vi "torque.vi"(5 "Optical":dbl, 6 "K":dbl=0.002, 7 "input_speed":dbl=905.26) -> (2 "Air gap distance":dbl, 3 "Torque":dbl format="%.5f")   [LabVIEW 2013]
panel:
  out "K 2":dbl
  in  "position":dbl[](array[numeric])=[0.006936158, 0.123434976, 0.06660524, 0.048499543, 0.042894394, 0.031233109, 0.017978293, -0.007572597, -0.007088973, -0.006314126, -0.013408862, -0.03698942, -0.059633605, -0.08709294, -0.061646755]
  in  "B":dbl[](array[numeric])=[361.6867357, 317.053774, 288.0813352, 251.2092617, 221.9672065, 202.0744938, 176.0201196, 159.6505095, 142.1246739, 127.4713834, 116.9721146, 102.8538267, 95.72786959, 84.33107726, 77.75646615]
  in  "Speed":dbl[](array[numeric])=[538.7343852, 571.7146956, 597.4120356, 616.9463637, 631.0607955, 641.0634852, 647.8692546, 652.8443821, 656.0759672, 658.4944862, 660.535588, 662.0915248, 663.3550631, 663.800211, 664.7743073]
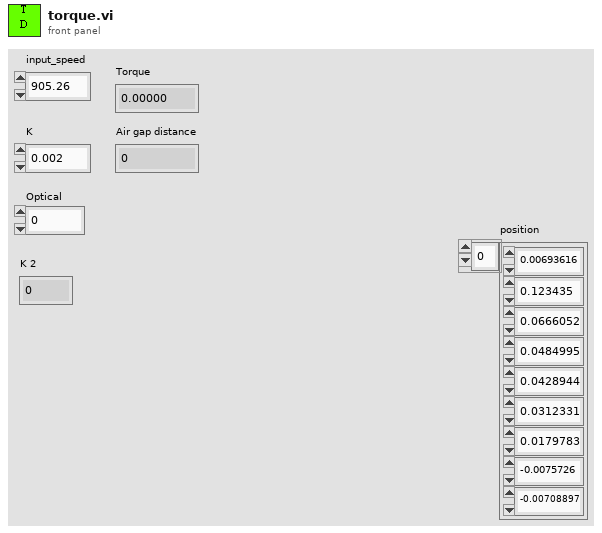
[diagram p1: front panel]
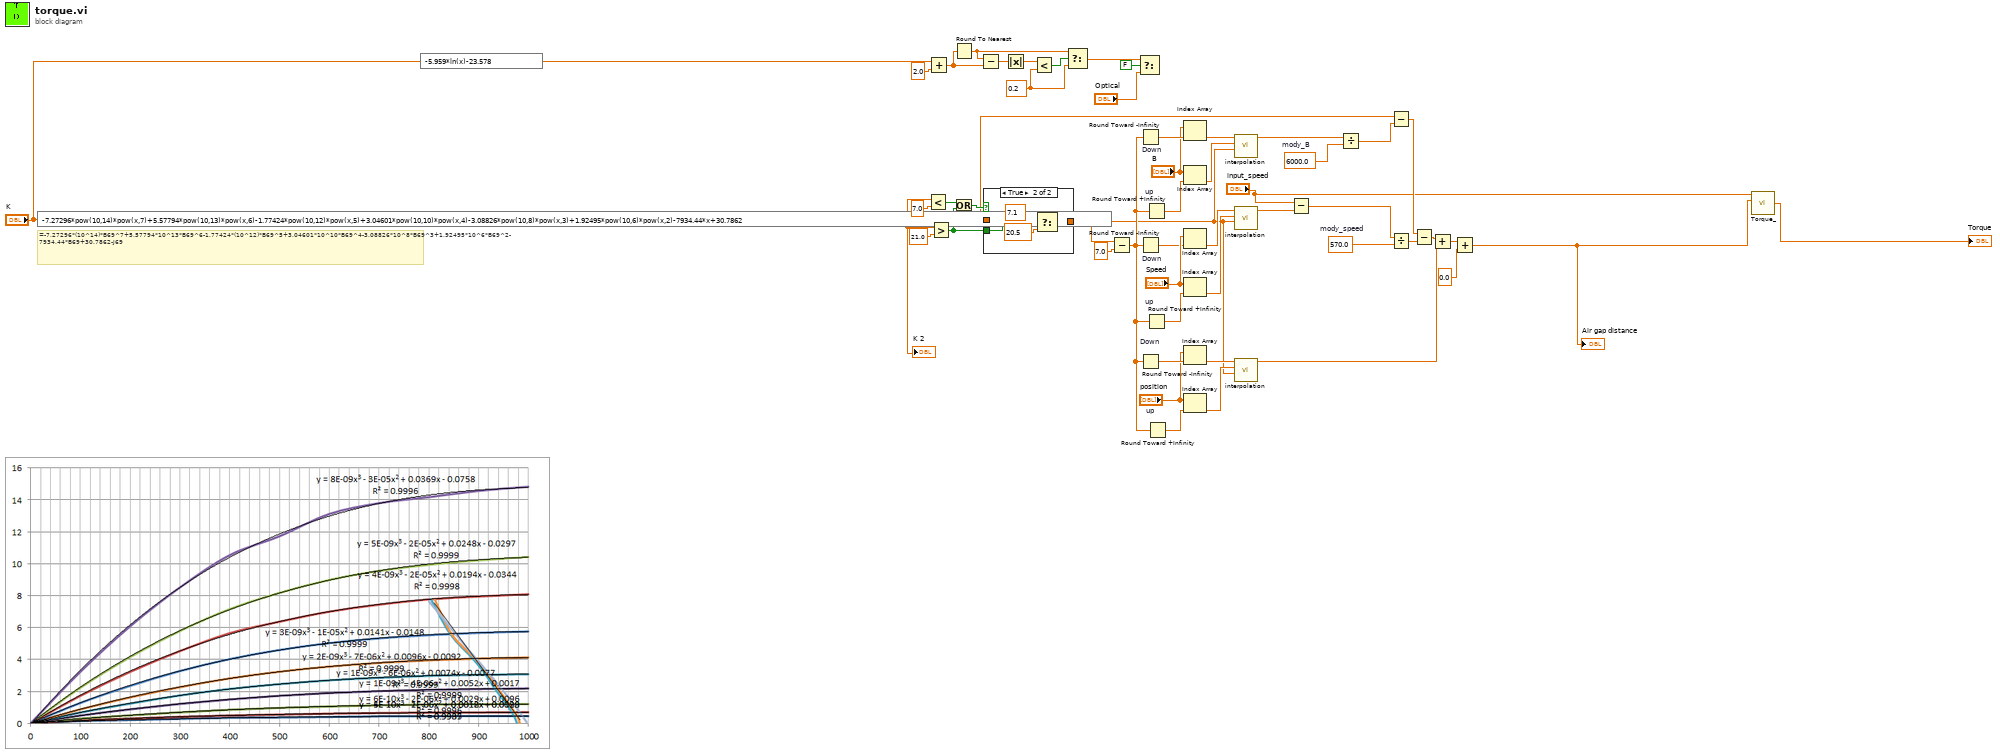
[diagram p0: block diagram]
diagram:
  w19 = 6000.0  # mody_B
  w26 = 570.0  # mody_speed
  w48 = 0.2 ("y")
  # "=-7.27296*(10^14)*B69^7+5.57794*10^13*B69^6-1.77424*(10^12)*B69^5+3.04601*10^10*B69^4-3.08826*10^8*B69^3+1.92495*10^6*B69^2-7934.44*B69+30.7862-J69"
  n1 = expression code="-7.27296*pow(10,14)*pow(x,7)+5.57794*pow(10,13)*pow(x,6)-1.77424*pow(10,12)*pow(x,5)+3.04601*pow(10,10)*pow(x,4)-3.08826*pow(10,8)*pow(x,3)+1.92495*pow(10,6)*pow(x,2)-7934.44*x+30.7862"("K") -> (w18:dbl)
  "K 2" <- w18
  n2 = expression code="-5.959*ln(x)-23.578"("K") -> (w47:dbl)
  n3 = Less?(x=w18, y=7.0) -> (x < y?=w35:bool)
  n4 = Add(x=w47, y=2.0) -> (x+y=w44:dbl)
  n5 = Greater?(x=w18, y=21.0) -> (0:w33:bool)
  n6 = Round To Nearest(number=w44) -> (nearest integer value=w45:dbl)
  n7 = Or(x=w35, y=w33) -> (x .or. y?=w34:bool)
  n8 = Subtract(x=w45, y=w44) -> (x-y=w51:dbl)
  n9 = case shown="True" w34 {
    tunnel: w18 -> [w52 _]
    tunnel: [w52 w54] -> w8
    tunnel: w33 -> [_ w56]
    frame False {
    }
    frame True {
      n10 = Select(t=7.1 ("K"), s=w56, f=20.5 ("K")) -> (s? t:f=w54:dbl)
    }
  }
  n11 = Absolute Value(x=w51) -> (abs(x)=w50:dbl)
  n12 = Less?(x=w50, y=w48) -> (x < y?=w49:bool)
  n13 = Select(t=w45, s=w49, f=w48) -> (s? t:f=w42:dbl)
  n14 = Subtract(x=w8, y=7.0) -> (x-y=w12:dbl)
  n15 = Select(t=w42, s=FALSE, f="Optical") -> ()  [unwired: 1 out]
  n16 = Round Toward -Infinity "Down"(1:w12) -> (0:w25:dbl)
  n17 = Round Toward -Infinity "Down"(1:w12) -> (0:w31:dbl)
  n18 = Round Toward -Infinity "Down"(1:w12) -> (0:w13:dbl)
  n19 = Round Toward +Infinity "up"(x=w12) -> (ceil(x): smallest int >= x=w24:dbl)
  n20 = Round Toward +Infinity "up"(x=w12) -> (ceil(x): smallest int >= x=w37:dbl)
  n21 = Round Toward +Infinity "up"(x=w12) -> (ceil(x): smallest int >= x=w14:dbl)
  n22 = Index Array(array="B", index=w25) -> (element=w22:dbl)
  n23 = Index Array(array="B", index=w24) -> (element=w21:dbl)
  n24 = Index Array(array="Speed", index=w31) -> (element=w29:dbl)
  n25 = Index Array(array="Speed", index=w37) -> (element=w30:dbl)
  n26 = Index Array(array="position", index=w13) -> (element=w10:dbl)
  n27 = Index Array(array="position", index=w14) -> (element=w9:dbl)
  n28 = call "interpolation.vi"("position"=w8, "Up"=w21, "Down"=w22) -> ("Output"=w20:dbl)  [unwired: 8 in]
  n29 = call "interpolation.vi"("position"=w8, "Up"=w30, "Down"=w29) -> ("Output"=w28:dbl)  [unwired: 8 in]
  n30 = call "interpolation.vi"("position"=w8, "Up"=w9, "Down"=w10) -> ("Output"=w6:dbl)  [unwired: 8 in]
  n31 = Subtract(x="input_speed", y=w28) -> (x-y=w27:dbl)
  n32 = Divide(x=w20, y=w19) -> (x/y=w17:dbl)
  n33 = Subtract(x=w18, y=w17) -> (x-y=w16:dbl)
  n34 = Divide(x=w27, y=w26) -> (x/y=w15:dbl)
  n35 = Subtract(x=w16, y=w15) -> (x-y=w7:dbl)
  n36 = Add(x=w7, y=w6) -> (x+y=w3:dbl)
  n37 = Add(x=w3, y=0.0) -> (x+y=w1:dbl)
  "Air gap distance" <- w1
  n38 = call "Torque_.vi"("gap"=w1, "input_speed"="input_speed") -> ("Torque"=→"Torque":dbl)  [unwired: 3 in, 1 out]
